vi "initializeCommunication.vi"(1 "Encoder COM Port":refnum<visa-resource-name>, 2 "Port":i32=1 min=1 max=255 step=1, 3 "Show Terminal":bool) -> (0 "Encoder VISA Resource Name (out)":refnum<visa-resource-name>)   [LabVIEW 2013]
panel:
  in  "Motor\nNumber":i32=1 min=1 max=4 step=1
  out "Port\nOpen\nStatus 2":bool
  out "Port\nOpen\nStatus":bool
  out "Motor Position":string
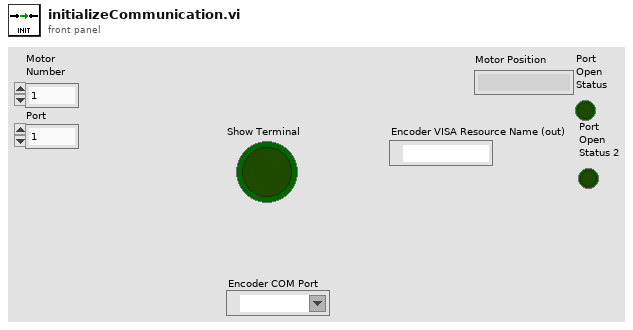
[diagram p1: front panel]
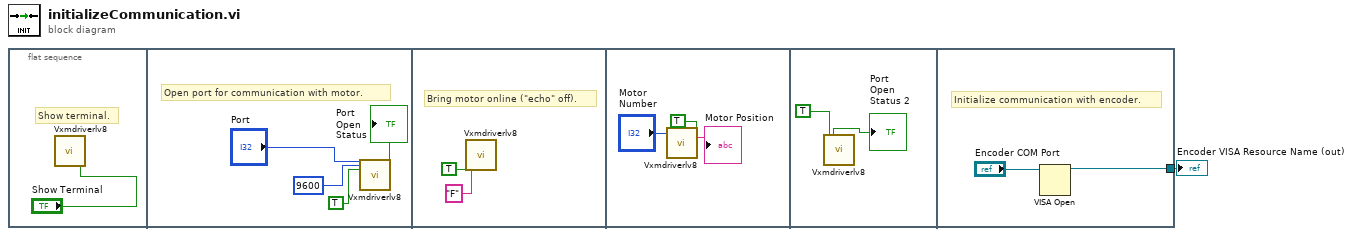
[diagram p0: block diagram]
diagram:
  n1 = flat-sequence {
    tunnel: [w15] -> w1
    frame #0 {
      # "Show terminal."
      n2 = call "Vxmdriverlv8.Vi"("Show Terminal"="Show Terminal") -> ()  [unwired: 21 in, 6 out]
    }
    frame #1 {
      # "Open port for communication with motor."
      n3 = call "Vxmdriverlv8.Vi"("Port"="Port", "Baud Rate"=9600, "Open Port"=TRUE) -> ("Port\nOpen\nStatus"=→"Port\nOpen\nStatus":bool)  [unwired: 19 in, 5 out]
    }
    frame #2 {
      # "Bring motor online (\"echo\" off)."
      n4 = call "Vxmdriverlv8.Vi"("Send\nchars\nto port"=TRUE ("Send\nchars\nto port"), "Chars to send"="F") -> ()  [unwired: 20 in, 6 out]
    }
    frame #3 {
      n5 = call "Vxmdriverlv8.Vi"("Get\nMotor\nPosition"=TRUE ("Get\nMotor\nPosition"), "Motor\nNumber"="Motor\nNumber") -> ("Motor Position"=→"Motor Position":string)  [unwired: 20 in, 5 out]
    }
    frame #4 {
      n6 = call "Vxmdriverlv8.Vi"("Is Port Open"=TRUE) -> ("Port\nOpen\nStatus"=→"Port\nOpen\nStatus 2":bool)  [unwired: 21 in, 5 out]
    }
    frame #5 {
      # "Initialize communication with encoder."
      n7 = VISA Open(VISA resource name="Encoder COM Port") -> (VISA resource name=w15:refnum<visa-resource-name>)  [unwired: 4 in, 1 out]
    }
  }
  "Encoder VISA Resource Name (out)" <- w1
